vi "TelemetryUpdate.vi"   [LabVIEW 2016]
uses:
  <vilib>/rvi/Emulation/niFpgaGetClockAttributes.vi
  <vilib>/rvi/Emulation/niFpgaSctlEmulationGetInTimedLoop.vi
  <vilib>/rvi/Emulation/niFpgaEmulationReportErrorSimple.vi
  <vilib>/rvi/Emulation/niFpgaEmulationIsFPGAContextNoSignature.vi
  <vilib>/rvi/errors/niFpgaSetErrorForExecOnDevCompSimple.vi
  <vilib>/rvi/eio/common/nirviEmuReportErrorAndStop.vi
  <vilib>/rvi/DataTransferAndStorage/Container/Common/niFpgaContainerGetUniqueNameForEmu.vi
  <vilib>/rvi/FIFO/Fifo_Resource/nirvififoEmulationSetSize.vi
  <vilib>/rvi/FIFO/Fifo_Resource/nirviFifoEmulationQueueMgr.vi
  <instcachedir>/0/nirviFifoEmulationQueueMgr_E5CAEC123FF24DC58D834DCA3CDAA9B5.lvgen/nirviFifoEmulationQueueMgr_E5CAEC123FF24DC58D834DCA3CDAA9B5_004.vi
  <vilib>/Utility/error.llb/Clear Errors.vi
  <vilib>/rvi/FIFO/Fifo_Resource/nirvififoEmulationCreateLock.vi
  <vilib>/rvi/Emulation/niFpgaProcessEmulError.vi
  <vilib>/rvi/FIFO/Fifo_Resource/nirvififoEmulationObtainLock.vi
  <vilib>/rvi/FIFO/Fifo_Resource/nirvififoEmulationReleaseLock.vi
  <vilib>/rvi/occurrence/nirviWaitOnOccurrenceBase.vi
  <vilib>/rvi/errors/nirviReportUnexpectedCaseInternalError.vi
  <vilib>/rvi/errors/nirviReportUnexpectedCaseInternalError (U32).vi
  <vilib>/rvi/Memory/Memory_Emulation/niFpgaMemoryEmulationCacheClearOnFirstRun.vi
  <vilib>/rvi/Memory/Memory_Emulation/nirvimemoryEmulationManagerCache_MakeExclusive.vi
  <vilib>/rvi/Memory/Memory_Emulation/niFpgaMemoryEmulationValidateCache.vi
  <vilib>/rvi/Memory/Memory_Emulation/nirvimemoryEmulationManagerCache_InsertValue.vi
  <vilib>/rvi/Memory/Memory_Emulation/nirvimemoryEmulationManagerCache_ReleaseExclusive.vi
  <vilib>/rvi/Memory/Memory_Emulation/nirvimemoryEmulationManagerCache_GetValue.vi
  <vilib>/rvi/Memory/Memory_Emulation/nirvimemoryEmulationManagerCache_SetValue.vi
  <vilib>/rvi/Emulation/niFpgaCriticalErrorInLSC.vi
  <vilib>/rvi/FIFO/Fifo_Resource/nirvififoEmulationDetermineInputValidOut.vi
  <vilib>/rvi/DataTransferAndStorage/Container/XNode/niFpgaContainer.xnode
  <vilib>/rvi/FIFO/Fifo_Resource/nirvififoEmulationRead.vi
  <vilib>/rvi/DataTransferAndStorage/Register/Emulation/niFpgaRegisterEmulation.vi
  <vilib>/rvi/FIFO/Fifo_Resource/nirvififoEmulationWrite.vi
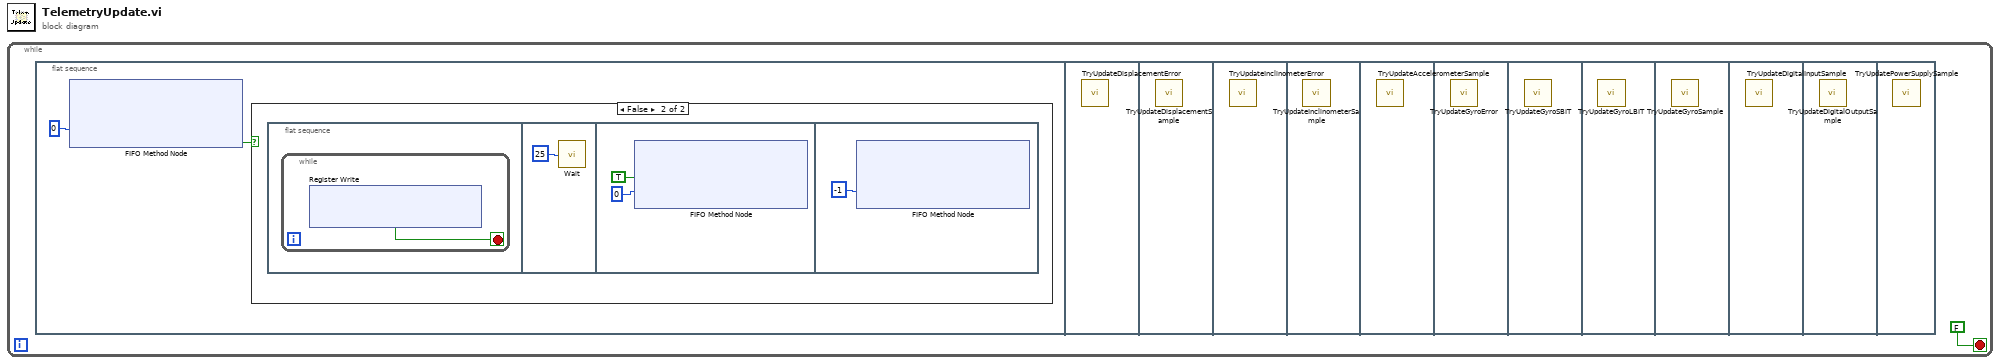
[diagram p0: block diagram]
diagram:
  n1 = while {
    stop <- FALSE stop-if-true
    n2 = flat-sequence {
      frame #0 {
        n3 = xnode ("FIFO Method Node")("Timeout"=0) -> ("Timed Out?"=w2:bool)  [unwired: 1 in, 2 out]
        n4 = case shown="False" w2 {
          frame True {
          }
          frame False {
            n5 = flat-sequence {
              frame #0 {
                n6 = while {
                  stop <- w4 stop-if-true
                  n7 = xnode "Register Write"() -> ("Data"=w4:bool)  [unwired: 1 in, 1 out]
                }
              }
              frame #1 {
                n8 = call "Wait"("Count(uSec)"=u8 25 ("Count(Ticks)")) -> ()  [unwired: 1 out]
              }
              frame #2 {
                n9 = xnode ("FIFO Method Node")("Element"=TRUE, "Timeout"=0) -> ()  [unwired: 1 in, 2 out]
              }
              frame #3 {
                n10 = xnode ("FIFO Method Node")("Timeout"=-1) -> ()  [unwired: 1 in, 3 out]
              }
            }
          }
        }
      }
      frame #1 {
        n11 = call "TryUpdateDisplacementError.vi"() -> ()  [unwired: 12 in]
      }
      frame #2 {
        n12 = call "TryUpdateDisplacementSample.vi"() -> ()  [unwired: 12 in]
      }
      frame #3 {
        n13 = call "TryUpdateInclinometerError.vi"() -> ()  [unwired: 12 in]
      }
      frame #4 {
        n14 = call "TryUpdateInclinometerSample.vi"() -> ()  [unwired: 12 in]
      }
      frame #5 {
        n15 = call "TryUpdateAccelerometerSample.vi"() -> ()  [unwired: 12 in]
      }
      frame #6 {
        n16 = call "TryUpdateGyroError.vi"() -> ()  [unwired: 12 in]
      }
      frame #7 {
        n17 = call "TryUpdateGyroSBIT.vi"() -> ()  [unwired: 12 in]
      }
      frame #8 {
        n18 = call "TryUpdateGyroLBIT.vi"() -> ()  [unwired: 12 in]
      }
      frame #9 {
        n19 = call "TryUpdateGyroSample.vi"() -> ()  [unwired: 12 in]
      }
      frame #10 {
        n20 = call "TryUpdateDigitalInputSample.vi"() -> ()  [unwired: 12 in]
      }
      frame #11 {
        n21 = call "TryUpdateDigitalOutputSample.vi"() -> ()  [unwired: 12 in]
      }
      frame #12 {
        n22 = call "TryUpdatePowerSupplySample.vi"() -> ()  [unwired: 12 in]
      }
    }
  }
